vi "SParam VST Calibration.vi"(8 "error in":errorcluster, 10 "RFmxVNA Settings":T2={"VST Resource Name"="VNA-5633", "RFSG Port"="", "RFmx Port"="", "RF Out Switch"="VNA-5633", "RF Out Connection"={"Common RFout"="", "Port1 Incident"="", "Port2 Incident"=""}, "RF In Switch"="VNA-5633", "RF In Connection"={"Common RFin"="", "Port1 Reference"="", "Port1 Test"="", "Port2 Reference"="", "Port2 Test"=""}, "RFSG attenuation mode"=enum."Constant Attenuation", "RFSG Constant Attenuation (dB)"=0.0, "Save Calibration File at"=path "", "Short S1P"=path "", "Open S1P"=path "", "Load S1P"=path "", "Through Adapter S2P"=path ""}, 11 "S-Par Reference In":T1) -> (0 "error out":errorcluster, 3 "S-Par Reference Out":T1)   [LabVIEW 2023]
uses:
  Controls/Hardware Config - SParam_VST.ctl
  <vilib>/niSPML/Typedefs/Session Handle.ctl
  <vilib>/niSPML/S-Par Reference.lvclass
  <vilib>/niSPML/S-parameters/Datatypes/S-Par Calibration Method.ctl
  <vilib>/niSPML/S-Parameter Measurements.lvlib
  <vilib>/niSPML/S-parameters/S-Parameters.lvlib
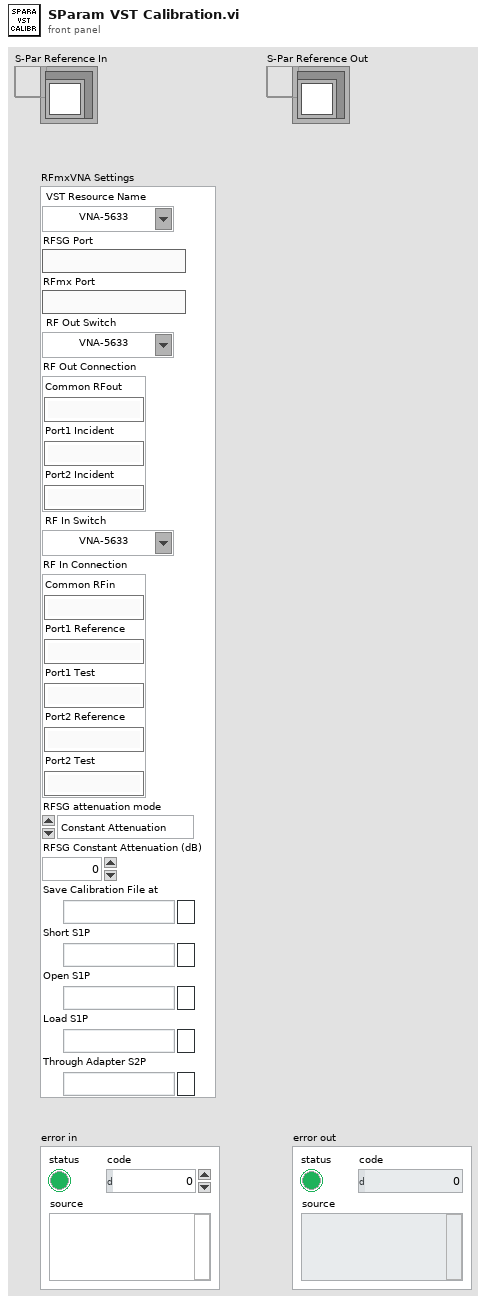
[diagram p1: front panel]
types:
  T1 = typedef "S-Parameter Measurements.lvlib/S-Par Reference.lvclass/Session Handle.ctl" = refnum<data-value>
  T2 = typedef "Hardware Config - SParam_VST.ctl" = cluster{"VST Resource Name":refnum<k15>, "RFSG Port":string, "RFmx Port":string, "RF Out Switch":refnum<k15>, "RF Out Connection":cluster{"Common RFout":string, "Port1 Incident":string, "Port2 Incident":string}, "RF In Switch":refnum<k15>, "RF In Connection":cluster{"Common RFin":string, "Port1 Reference":string, "Port1 Test":string, "Port2 Reference":string, "Port2 Test":string}, "RFSG attenuation mode":enum32{"<None>", "Constant Attenuation"}, "RFSG Constant Attenuation (dB)":dbl, "Save Calibration File at":path, "Short S1P":path, "Open S1P":path, "Load S1P":path, "Through Adapter S2P":path}
  T3 = typedef "S-Parameters.lvlib/S-Par Calibration Method.ctl" = i32
  T4 = typedef "S-Parameter Measurements.lvlib/LString Handle Array.ctl" = string[]
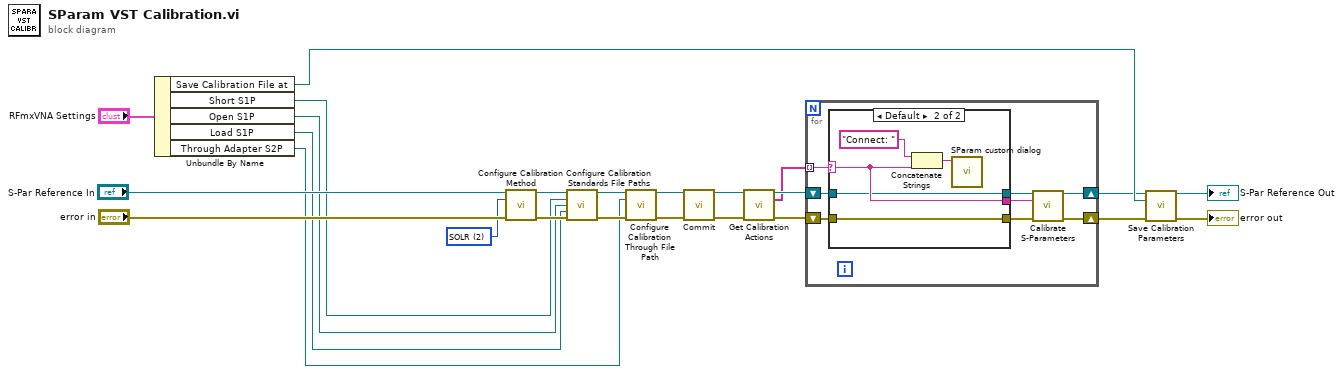
[diagram p0: block diagram]
diagram:
  w1 = T3 2 items=["None", "QSOLT", "SOLR", "SOLT", "Thru"] ("Calibration Method")
  n1 = Unbundle By Name("RFmxVNA Settings") -> ("Save Calibration File at"=w9:path, "Short S1P"=w10:path, "Open S1P"=w11:path, "Load S1P"=w12:path, "Through Adapter S2P"=w13:path)
  n2 = call <vilib>:"Configure Calibration Method.vi"("S-Par Reference In"="S-Par Reference In", "Calibration Method"=w1, "error in"="error in") -> ("S-Par Reference Out"=w20:T1, "error out"=w19:errorcluster)  [unwired: 11 in]
  n3 = call <vilib>:"Configure Calibration Standards File Paths.vi"("S-Par Reference In"=w20, "Short s1p File Path"=w10, "Open s1p File Path"=w11, "Load s1p File Path"=w12, "error in"=w19) -> ("S-Par Reference Out"=w22:T1, "error out"=w21:errorcluster)  [unwired: 9 in]
  n4 = call <vilib>:"Configure Calibration Through File Path.vi"("S-Par Reference In"=w22, "Through s2p File Path"=w13, "error in"=w21) -> ("S-Par Reference Out"=w18:T1, "error out"=w17:errorcluster)  [unwired: 11 in]
  n5 = call <vilib>:"Commit.vi"("S-Par Reference In"=w18, "error in"=w17) -> ("S-Par Reference Out"=w24:T1, "error out"=w23:errorcluster)  [unwired: 12 in]
  n6 = call <vilib>:"Get Calibration Actions.vi"("S-Par Reference In"=w24, "error in"=w23) -> ("S-Par Reference Out"=w8:T1, "Calibration Actions"=w6:T4, "error out"=w7:errorcluster)  [unwired: 11 in]
  n7 = for {
    shift-right: [w32] -> w5
    shift-left: w8 -> [w27]
    shift-right: [w31] -> w4
    shift-left: w7 -> [w25]
    tunnel: w6 -> [w30] mode=indexing
    n8 = case shown="Default" w30 {
      selector: w30 -> [w35 w39]
      tunnel: [w35 w39] -> w29
      tunnel: [w33 w38] -> w28
      tunnel: w27 -> [w33 w38]
      tunnel: [w34 w36] -> w26
      tunnel: w25 -> [w34 w36]
      frame "Calculate" {
      }
      frame Default {
        n9 = Concatenate Strings("Connect: " ("string"), w39) -> (w37:string)
        n10 = call "SParam custom dialog.vi"("Message"=w37) -> ()  [unwired: 11 in]
      }
    }
    n11 = call <vilib>:"Calibrate S-Parameters.vi"("S-Par Reference In"=w28, "Calibration Action"=w29, "error in"=w26) -> ("S-Par Reference Out"=w32:T1, "error out"=w31:errorcluster)  [unwired: 11 in]
  }
  n12 = call <vilib>:"Save Calibration Parameters.vi"("S-Par Reference In"=w5, "Calibration Parameters File Path"=w9, "error in"=w4) -> ("S-Par Reference Out"=→"S-Par Reference Out":T1, "error out"=→"error out":errorcluster)  [unwired: 11 in]
